vi "Manipulator Controller.vi"   [LabVIEW 2018]
uses:
  <vilib>/Rock Robotics/WPI/Joystick/WPI_JoystickDeviceEnum.ctl
  Manipulator Controller Global.vi
types:
  T1 = typedef "WPI_JoystickDeviceEnum.ctl" = enum16{"USB 0", "USB 1", "USB 2", "USB 3", "USB 4", "USB 5"}
  T2 = typedef "WPI_JoystickDevRef.ctl" = cluster{"Device":T1}
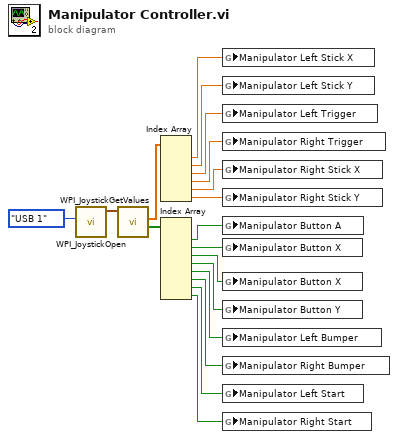
[diagram p0: block diagram]
diagram:
  n1 = call <vilib>:"WPI_JoystickOpen.vi"("JoystickDevice"=WPI_JoystickDeviceEnum."USB 1") -> ("JoystickDevRef"=w17:T2)  [unwired: 10 in]
  n2 = call <vilib>:"WPI_JoystickGetValues.vi"("JoystickDevRef"=w17) -> ("Buttons"=w15:bool[], "Axes"=w16:dbl[])  [unwired: 6 in, 3 out]
  n3 = Index Array(array=w16) -> (element #1=w14:dbl, element #2=w13:dbl, element #3=w12:dbl, element #4=w11:dbl, element #5=w10:dbl, element #6=w9:dbl)  [unwired: 6 in]
  n4 = Index Array(array=w15) -> (element #1=w8:bool, element #2=w7:bool, element #3=w6:bool, element #4=w5:bool, element #5=w4:bool, element #6=w3:bool, element #7=w2:bool, element #8=w1:bool)  [unwired: 8 in]
  n5 = global write "Manipulator Controller Global.vi" "Manipulator Left Stick X"(w14) -> ()
  n6 = global write "Manipulator Controller Global.vi" "Manipulator Left Stick Y"(w13) -> ()
  n7 = global write "Manipulator Controller Global.vi" "Manipulator Left Trigger"(w12) -> ()
  n8 = global write "Manipulator Controller Global.vi" "Manipulator Right Trigger"(w11) -> ()
  n9 = global write "Manipulator Controller Global.vi" "Manipulator Right Stick X"(w10) -> ()
  n10 = global write "Manipulator Controller Global.vi" "Manipulator Right Stick Y"(w9) -> ()
  n11 = global write "Manipulator Controller Global.vi" "Manipulator Button A"(w8) -> ()
  n12 = global write "Manipulator Controller Global.vi" "Manipulator Button X"(w7) -> ()
  n13 = global write "Manipulator Controller Global.vi" "Manipulator Button X"(w6) -> ()
  n14 = global write "Manipulator Controller Global.vi" "Manipulator Button Y"(w5) -> ()
  n15 = global write "Manipulator Controller Global.vi" "Manipulator Left Bumper"(w4) -> ()
  n16 = global write "Manipulator Controller Global.vi" "Manipulator Right Bumper"(w3) -> ()
  n17 = global write "Manipulator Controller Global.vi" "Manipulator Left Start"(w2) -> ()
  n18 = global write "Manipulator Controller Global.vi" "Manipulator Right Start"(w1) -> ()
